vi "Fill ActorsRef Container.vi"(7 "Mode":enum16{"Modules", "Logs"}(ring), 8 "error in (no error)":errorcluster, 10 "Ref Data Object":refnum<class "ActorRefContainer.lvclass">, 11 "Core In":refnum<class "Core.lvclass">) -> (0 "error out":errorcluster, 3 "Core Out":refnum<class "Core.lvclass">)   [LabVIEW 2019, in "Core.lvlib" / "Core.lvclass"]
uses:
  Core.lvclass
  C:/Projekty/_Wewnetrzne/PC_ActorFramework/07_Program/LABVIEW/02_Source/Modules/ModuleAbstract/ModuleAbstract.lvclass
  Containers/ActorRefContainer/ActorRefContainer.lvclass
  Containers/ActorRefContainer/ActorRefContainer.lvclass/ActorRefContainer.ctl
  ModuleAbstract/ModuleAbstract.lvclass/ModuleAbstract.ctl
  <vilib>/ActorFramework/Message Enqueuer/Message Enqueuer.lvclass
  6b19e6b0-dc0c-4aed-ac36-1c1cf044dd47.vi
  bf18d584-55da-42a1-abbe-36702a541740.vi
  Containers/ActorRefContainer/Accessors/ActorRefContainer Write Modules.vi
  6b19e6b0-dc0c-4aed-ac36-1c1cf044dd47.vi/c26b3069-90c9-40c4-8ed2-b9b8c41aca42.vi
  bf18d584-55da-42a1-abbe-36702a541740.vi/094d3b59-bbeb-40d8-8175-fe143e6e0a0d.vi
  Containers/ActorRefContainer/Accessors/ActorRefContainer Write Logs.vi
  <userlib>/_OpenG.lib/lvdata/lvdata.llb/Array to VCluster__ogtk.vi
  ModuleAbstract/ModuleAbstract.lvclass
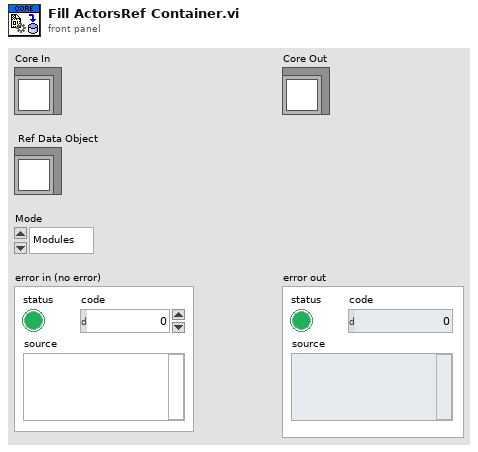
[diagram p1: front panel]
types:
  T1 = cluster{"ModuleRef":refnum<class "Message Enqueuer.lvclass">, "UIRef":refnum<class "Message Enqueuer.lvclass">}
  T2 = cluster{"Core":cluster{"ModuleRef":refnum<class "Message Enqueuer.lvclass">, "UIRef":refnum<class "Message Enqueuer.lvclass">}}
  T3 = cluster{"Core":cluster{"ModRef":refnum<class "Message Enqueuer.lvclass">, "UIRef":refnum<class "Message Enqueuer.lvclass">}}
  T4 = cluster{"EventLog":cluster{"ModRef":refnum<class "Message Enqueuer.lvclass">, "UIRef":refnum<class "Message Enqueuer.lvclass">}}
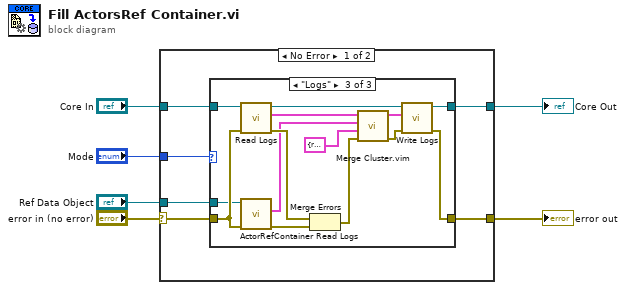
[diagram p0: block diagram]
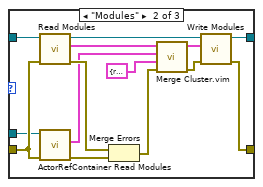
[diagram p3: hidden frame]
diagram:
  n1 = case shown="No Error" "error in (no error)" {
    selector: "error in (no error)" -> [w7 w44]
    tunnel: [w12 w44] -> w6
    tunnel: "Mode" -> [w11 _]
    tunnel: [w10 w43] -> w4
    tunnel: "Core In" -> [w9 w43]
    tunnel: "Ref Data Object" -> [w8 _]
    frame No Error {
      n2 = case shown="\"Logs\"" w11 {
        tunnel: w7 -> [w13 w28 w42]
        tunnel: w8 -> [_ w27 w41]
        tunnel: w9 -> [w14 w26 w40]
        tunnel: [w14 w17 w31] -> w10
        tunnel: [w13 w16 w30] -> w12
        frame Default {
        }
        frame "Modules" {
          n3 = call "Read Modules.vi"("error in (no error)"=w28, "ModuleAbstract in"=w26) -> ("error out"=w24:errorcluster, "Modules"=w21:T2, "ModuleAbstract out"=w18:refnum<class "Core.lvclass">)  [unwired: 7 in]
          n4 = call "ActorRefContainer Read Modules.vi"("error in (no error)"=w28, "ActorRefContainer in"=w27) -> ("error out"=w25:errorcluster, "Modules"=w23:T3)  [unwired: 7 in, 1 out]
          n5 = Merge Errors(w24, w25) -> (w22:errorcluster)
          n6 = call "Merge Cluster.vim"("error in (no error)"=w22, "Default Element"=T1 {"ModuleRef"=refnum, "UIRef"=refnum}, "Claster to Merge"=w23, "Main Cluster"=w21) -> ("error out"=w19:errorcluster, "Merged Main Cluster"=w20:T2)  [unwired: 6 in]
          n7 = call "Write Modules.vi"("error in (no error)"=w19, "Modules"=w20, "ModuleAbstract in"=w18) -> ("error out"=w16:errorcluster, "ModuleAbstract out"=w17:refnum<class "Core.lvclass">)  [unwired: 7 in]
        }
        frame "Logs" {
          n8 = call "Read Logs.vi"("error in (no error)"=w42, "ModuleAbstract in"=w40) -> ("error out"=w38:errorcluster, "Logs"=w35:T4, "ModuleAbstract out"=w32:refnum<class "Core.lvclass">)  [unwired: 7 in]
          n9 = call "ActorRefContainer Read Logs.vi"("error in (no error)"=w42, "ActorRefContainer in"=w41) -> ("error out"=w39:errorcluster, "Logs"=w37:T4)  [unwired: 7 in, 1 out]
          n10 = Merge Errors(w38, w39) -> (w36:errorcluster)
          n11 = call "Merge Cluster.vim"("error in (no error)"=w36, "Default Element"=T1 {"ModuleRef"=refnum, "UIRef"=refnum}, "Claster to Merge"=w37, "Main Cluster"=w35) -> ("error out"=w33:errorcluster, "Merged Main Cluster"=w34:T4)  [unwired: 6 in]
          n12 = call "Write Logs.vi"("error in (no error)"=w33, "Logs"=w34, "ModuleAbstract in"=w32) -> ("error out"=w30:errorcluster, "ModuleAbstract out"=w31:refnum<class "Core.lvclass">)  [unwired: 7 in]
        }
      }
    }
    frame Error {
    }
  }
  "error out" <- w6
  "Core Out" <- w4
